vi "Pre Loop Action.vi"(8 "error in":errorcluster, 11 "Ref In":refnum<vi>) -> (0 "error out":errorcluster, 2 "Module Data Out":refnum<class "Rename.lvclass">, 3 "Stop Event Refnum":refnum<event-registration>)   [LabVIEW 2015, in "Generic Module Library.lvlib" / "Template G_Module.lvlib"]
uses:
  Template G_Module.lvlib
  Private Controls/Module Message Cluster.ctl
  Module Class/Rename.lvclass
  Module Communications/Queue Support/Queue Reference Actions.ctl
  Private Controls/Module Message Cluster Components/Acknowledge Data Cluster.ctl
  Private Controls/Module Message Cluster Components/Message Data Cluster.ctl
  Module Broadcasts/Broadcast Support/Broadcast Actions.ctl
  Private Controls/Event Item.ctl
  Module Broadcasts/API/Broadcast List.ctl
  Module Broadcasts/Broadcast Support/Registration Actions.ctl
  Private Controls/Module Message Cluster Components/Ack Payload.ctl
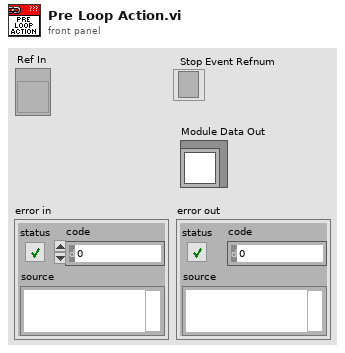
[diagram p1: front panel]
types:
  T1 = typedef "Generic Module Library.lvlib/Template G_Module.lvlib/Registration Actions.ctl" = enum16{"Create", "Get", "Destroy"}
  T2 = typedef "Generic Module Library.lvlib/Template G_Module.lvlib/Broadcast List.ctl" = cluster{"Module Started":refnum<user-event>, "Module Error":refnum<user-event>, "Module Pong":refnum<user-event>, "Module Status":refnum<user-event>, "Module Stopping":refnum<user-event>, "Module Stopped":refnum<user-event>, "Module Reinitialized":refnum<user-event>}
  T3 = typedef "Generic Module Library.lvlib/Template G_Module.lvlib/Broadcast Actions.ctl" = enum16{"Create", "Get", "Destroy"}
  T4 = typedef "Generic Module Library.lvlib/Template G_Module.lvlib/Queue Reference Actions.ctl" = enum16{"Release", "Set", "Get"}
  T5 = typedef "Generic Module Library.lvlib/Template G_Module.lvlib/Module Message Cluster.ctl" = cluster{"Message Data":T6, "Acknowledge Data":T7}
  T6 = typedef "Generic Module Library.lvlib/Template G_Module.lvlib/Message Data Cluster.ctl" = cluster{"Module Action":string, "Message Data":variant}
  T7 = typedef "Generic Module Library.lvlib/Template G_Module.lvlib/Acknowledge Data Cluster.ctl" = cluster{"Ack Requested":bool, "Ack Notifier Ref":refnum<notifier>, "Response Payload":T8}
  T8 = typedef "Generic Module Library.lvlib/Template G_Module.lvlib/Ack Payload.ctl" = cluster{"Response Data":string, "error out":errorcluster}
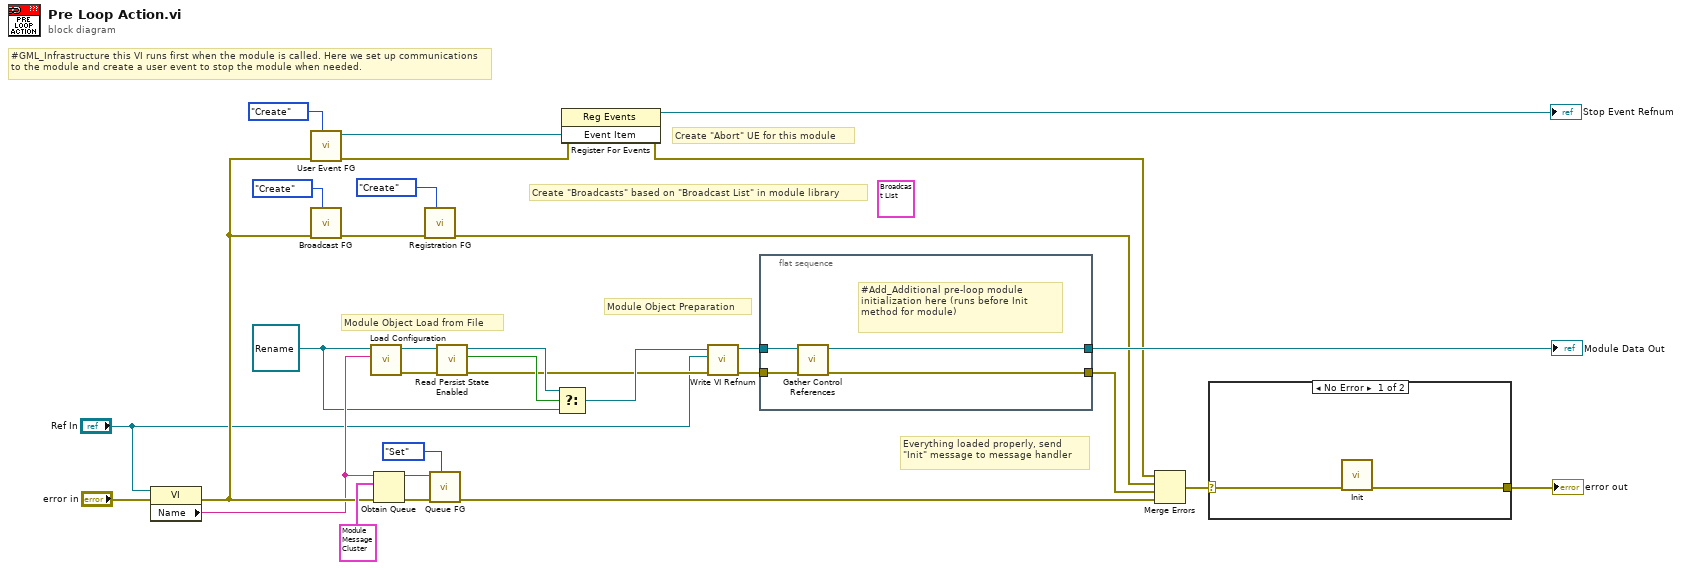
[diagram p0: block diagram]
diagram:
  (unwired) T2 {"Module Started"=refnum, "Module Error"=refnum, "Module Pong"=refnum, "Module Status"=refnum, "Module Stopping"=refnum, "Module Stopped"=refnum, "Module Reinitialized"=refnum} ("Broadcast List")
  w3 = refnum<class "Rename.lvclass"> refnum ("Generic Module Library.lvlib:Template Module.lvlib:Rename.lvclass")
  # "Module Object Load from File"
  # "Everything loaded properly, send \"Init\" message to message handler"
  # "Create \"Broadcasts\" based on \"Broadcast List\" in module library"
  # "#GML_Infrastructure this VI runs first when the module is called. Here we set up communications to the module and create a user event to stop the module when needed."
  # "Module Object Preparation"
  # "Create \"Abort\" UE for this module"
  n1 = property on="Property Node" class="VI"(reference="Ref In", error in="error in") -> (error out=w15:errorcluster, "Name"=w14:string)  [unwired: 1 out]
  n2 = call "User Event FG.vi"("User Event Actions"=enum16{"Destroy", "Create", "Get"}."Create", "error in"=w15) -> ("error out"=w26:errorcluster, "Event Item"=w28:refnum<user-event>)  [unwired: 8 in]
  n3 = call "Broadcast FG.vi"("Broadcast Actions"=Broadcast_Actions."Create", "error in"=w15) -> ("error out"=w18:errorcluster)  [unwired: 8 in, 1 out]
  n4 = call "Load Configuration.vi"("Module Name"=w14, "Module Data In"=w3) -> ("error out"=w6:errorcluster, "Module Data Out"=w7:refnum<class "Rename.lvclass">)  [unwired: 8 in]
  n5 = Obtain Queue(name (unnamed)=w14, element data type=T5 {"Message Data"={"Module Action"="", "Message Data"=variant}, "Acknowledge Data"={"Ack Requested"=FALSE, "Ack Notifier Ref"=refnum, "Response Payload"={"Response Data"="", "error out"={"status"=FALSE, "code"=0, "source"=""}}}} ("Module Message Cluster"), error in (no error)=w15) -> (queue out=w30:refnum<queue>, error out=w29:errorcluster)  [unwired: 2 in, 1 out]
  n6 = call "Registration FG.vi"("Registration Actions"=Registration_Actions."Create", "error in"=w18) -> ("error out"=w13:errorcluster)  [unwired: 8 in, 1 out]
  n7 = call "Queue FG.vi"("Queue Reference Actions"=Queue_Reference_Actions."Set", "error in"=w29, "Queue in"=w30) -> ("error out"=w11:errorcluster)  [unwired: 7 in, 1 out]
  n8 = call-dynamic "Read Persist State Enabled.vi"("error in (no error)"=w6, "Rename in"=w7) -> ("error out"=w2:errorcluster, "Persist State Enabled"=w5:bool, "Rename out"=w4:refnum<class "Rename.lvclass">)  [unwired: 7 in]
  n9 = Select(t=w4, s=w5, f=w3) -> (s? t:f=w8:refnum<class "Rename.lvclass">)
  n10 = register-events(error in=w26, w28) -> (reference out=→"Stop Event Refnum":refnum<event-registration>, error out=w20:errorcluster)  [unwired: 1 in]
  n11 = call-dynamic "Write VI Refnum.vi"("error in (no error)"=w2, "VI Refnum"="Ref In", "Module Data In"=w8) -> ("error out"=w17:errorcluster, "Module Data Out"=w16:refnum<class "Rename.lvclass">)  [unwired: 7 in]
  n12 = flat-sequence {
    tunnel: [w32] -> w23
    tunnel: [w33] -> w22
    tunnel: w16 -> [w35]
    tunnel: w17 -> [w34]
    frame #0 {
      # "#Add_Additional pre-loop module initialization here (runs before Init method for module)"
      n13 = call "Gather Control References.vi"("error in (no error)"=w34, "Rename in"=w35) -> ("error out"=w33:errorcluster, "Rename out"=w32:refnum<class "Rename.lvclass">)  [unwired: 8 in]
    }
  }
  n14 = Merge Errors(w20, w13, w22, w11) -> (w9:errorcluster)
  n15 = case shown="No Error" w9 {
    selector: w9 -> [w36 w38]
    tunnel: [w37 w38] -> w10
    frame No Error {
      n16 = call "Init.vi"("error in"=w36) -> ("error out"=w37:errorcluster)  [unwired: 10 in]
    }
    frame Error {
    }
  }
  "error out" <- w10
  "Module Data Out" <- w23
